vi "QTrkGetDebugImage.vi"(8 "error in (no error)":errorcluster, 10 "id":i32, 11 "QTrk Instance":T1) -> (0 "error out":errorcluster, 1 "data":sgl[][](array[numeric]), 3 "QTrk Instance (out)":T1)   [LabVIEW 2011]
uses:
  QTrkInstance.ctl
  QTrkDLL.vi
panel:
  in  "image":sgl[][](array[numeric])
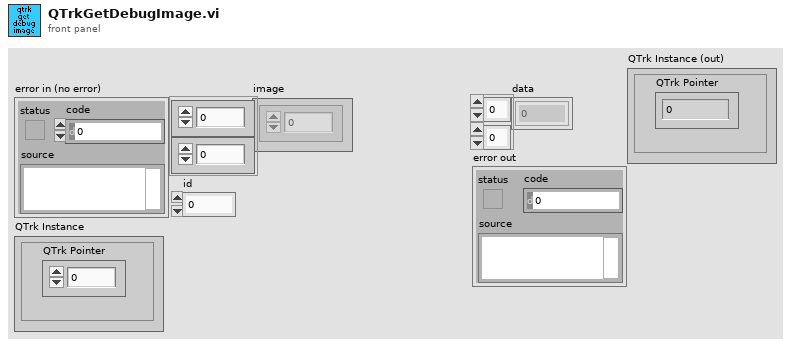
[diagram p1: front panel]
types:
  T1 = typedef "QTrkInstance.ctl" = cluster{"QTrk Pointer":u64}
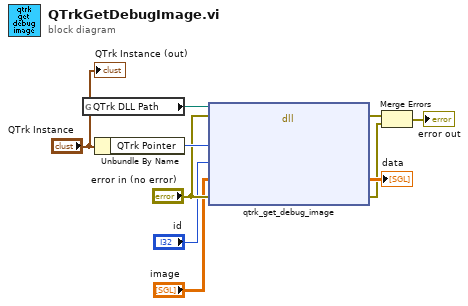
[diagram p0: block diagram]
diagram:
  n1 = global read "QTrkDLL.vi" "QTrk DLL Path"() -> (w10:path)
  n2 = Unbundle By Name("QTrk Instance") -> ("QTrk Pointer"=w8:u64)
  n3 = dll-call lib="D:/jcnossen1/cudaqi-tracker/bin/jtrk-labview.dll" fn="qtrk_get_debug_image"(path in=w10, error in="error in (no error)", "tracker"=w8, "id"="id", "data"="image", "error"="error in (no error)") -> (error out=w3:errorcluster, "data"=→"data":sgl[][], "error"=w2:errorcluster)  [unwired: 4 in, 1 out]
  n4 = Merge Errors(w3, w2) -> (→"error out":errorcluster)
  "QTrk Instance (out)" <- "QTrk Instance"
